vi "BallCalc.vi"(0 "Camera Angle (Rad)":dbl format="%#_13g", 1 "Object Viewport Width (px)":dbl) -> (2 "Target Distance (in)":dbl, 3 "Angle (deg, from vertical)":dbl format="%#_13g", 4 "Target RPM":dbl format="%#_13g")   [LabVIEW 2015]
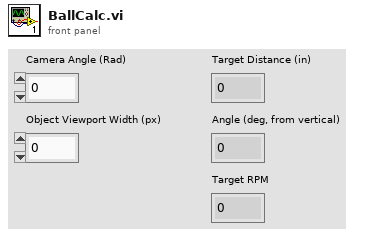
[diagram p1: front panel]
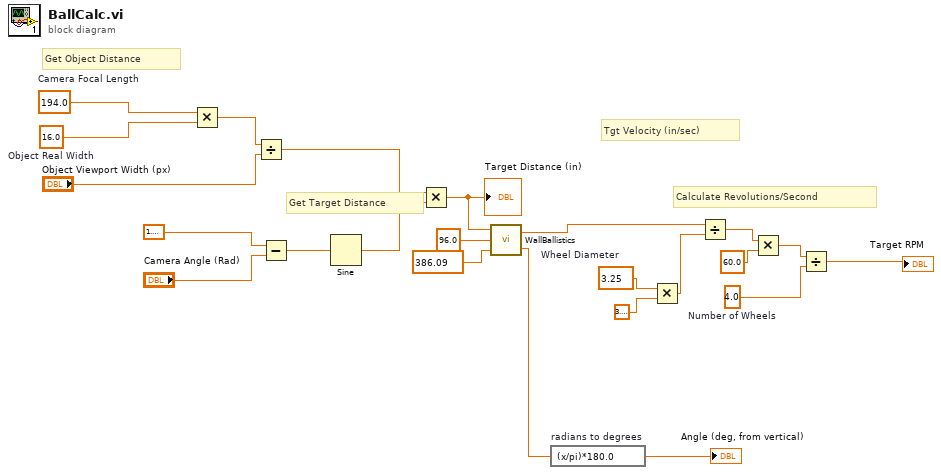
[diagram p0: block diagram]
diagram:
  w12 = 4.0  # Number of Wheels
  w15 = 3.25  # Wheel Diameter
  w22 = 16.0  # Object Real Width
  w23 = 194.0  # Camera Focal Length
  # "Tgt Velocity (in/sec)"
  # "Calculate Revolutions/Second"
  # "Get Target Distance"
  # "Get Object Distance"
  n1 = Multiply(x=w23, y=w22) -> (x*y=w21:dbl)
  n2 = Divide(x=w21, y="Object Viewport Width (px)") -> (x/y=w7:dbl)
  n3 = Subtract(x=1.5707963267948966, y="Camera Angle (Rad)") -> (x-y=w17:dbl)
  n4 = Sine(x=w17) -> (sin(x)=w6:dbl)
  n5 = Multiply(x=w7, y=w6) -> (x*y=w5:dbl)
  "Target Distance (in)" <- w5
  n6 = call "WallBallistics.vi"("Gravitational Constant"=386.09, "Object Y Offset"=96.0, "Target Distance"=w5) -> ("Angle (Radians)"=w1:dbl, "Velocity"=w2:dbl)
  n7 = expression code="(x/pi)*180.0" "radians to degrees"(w1) -> (→"Angle (deg, from vertical)":dbl)
  n8 = Multiply(x=w15, y=3.141592653589793) -> (x*y=w13:dbl)
  n9 = Divide(x=w2, y=w13) -> (x/y=w9:dbl)
  n10 = Multiply(x=w9, y=60.0) -> (x*y=w11:dbl)
  n11 = Divide(x=w11, y=w12) -> (x/y=→"Target RPM":dbl)
